vi "Collect_Indexes_for_Jumps-3.vi"(4 "[IN] # Track with \nThird Problem Point":i32, 5 "[IN] Index of Third\nProblem point":i32, 6 "[IN] # Track with \nSecond Problem Point":i32, 7 "[IN] Index of Point Be\nfore Problem (Origin)":i32, 8 "[IN] Index of Second\nProblem point":i32, 9 "[IN] # Track with First\nProblem Point":i32, 10 "[IN] Index of First \nProblem Point":i32, 11 "[IN] # Track of Origin":i32) -> (1 "[OUT] Indexes for Jumps":i32[](array[numeric]))   [LabVIEW 2017]
doc: "The subVI constructs the array with indicies of all problem points"
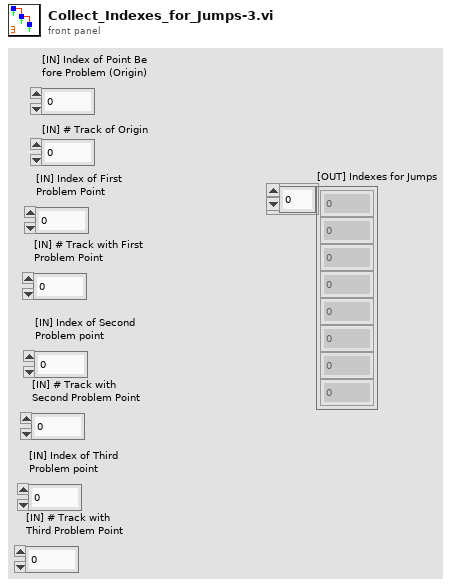
[diagram p1: front panel]
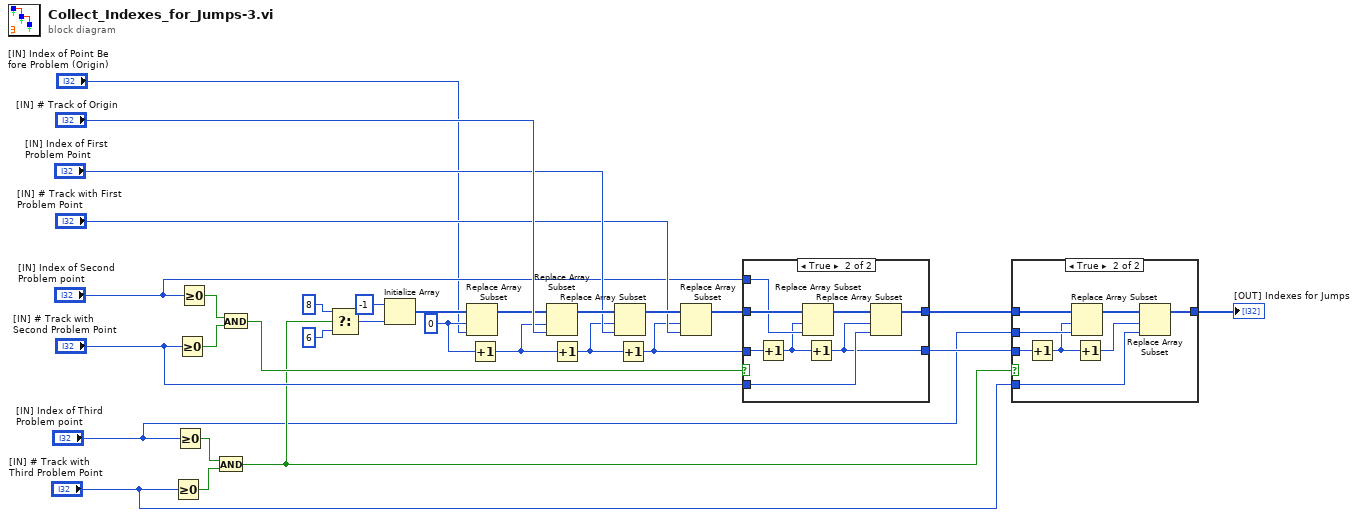
[diagram p0: block diagram]
diagram:
  w11 = 0
  n1 = Greater Or Equal To 0?(x="[IN] # Track with \nThird Problem Point") -> (x >= 0?=w8:bool)
  n2 = Greater Or Equal To 0?(x="[IN] Index of Third\nProblem point") -> (x >= 0?=w7:bool)
  n3 = Greater Or Equal To 0?(x="[IN] # Track with \nSecond Problem Point") -> (x >= 0?=w28:bool)
  n4 = Greater Or Equal To 0?(x="[IN] Index of Second\nProblem point") -> (x >= 0?=w29:bool)
  n5 = And(x=w7, y=w8) -> (x .and. y?=w4:bool)
  n6 = And(x=w29, y=w28) -> (x .and. y?=w18:bool)
  n7 = Select(t=8, s=w4, f=6) -> (s? t:f=w25:i32)
  n8 = Initialize Array(-1 ("[IN] # Track of Origin"), w25) -> (w13:i32[])
  n9 = Replace Array Subset(array=w13, new element="[IN] Index of Point Be\nfore Problem (Origin)", index=w11) -> (w12:i32[])
  n10 = Increment(x=w11) -> (x+1=w9:i32)
  n11 = Replace Array Subset(array=w12, new element="[IN] # Track of Origin", index=w9) -> (w23:i32[])
  n12 = Increment(x=w9) -> (x+1=w21:i32)
  n13 = Replace Array Subset(array=w23, new element="[IN] Index of First \nProblem Point", index=w21) -> (w20:i32[])
  n14 = Increment(x=w21) -> (x+1=w16:i32)
  n15 = Replace Array Subset(array=w20, new element="[IN] # Track with First\nProblem Point", index=w16) -> (w17:i32[])
  n16 = case shown="True" w18 {
    tunnel: w17 -> [w32 w40]
    tunnel: w16 -> [w31 w39]
    tunnel: "[IN] Index of Second\nProblem point" -> [_ w38]
    tunnel: "[IN] # Track with \nSecond Problem Point" -> [_ w35]
    tunnel: [w32 w34] -> w6
    tunnel: [w31 w33] -> w5
    frame False {
    }
    frame True {
      n17 = Increment(x=w39) -> (x+1=w36:i32)
      n18 = Replace Array Subset(array=w40, new element=w38, index=w36) -> (w37:i32[])
      n19 = Increment(x=w36) -> (x+1=w33:i32)
      n20 = Replace Array Subset(array=w37, new element=w35, index=w33) -> (w34:i32[])
    }
  }
  n21 = case shown="True" w4 {
    tunnel: w6 -> [w41 w49]
    tunnel: w5 -> [_ w48]
    tunnel: "[IN] Index of Third\nProblem point" -> [_ w47]
    tunnel: "[IN] # Track with \nThird Problem Point" -> [_ w43]
    tunnel: [w41 w42] -> w1
    frame False {
    }
    frame True {
      n22 = Increment(x=w48) -> (x+1=w45:i32)
      n23 = Replace Array Subset(array=w49, new element=w47, index=w45) -> (w46:i32[])
      n24 = Increment(x=w45) -> (x+1=w44:i32)
      n25 = Replace Array Subset(array=w46, new element=w43, index=w44) -> (w42:i32[])
    }
  }
  "[OUT] Indexes for Jumps" <- w1
